vi "Initialize.vi"(8 "error in (no error)":errorcluster, 11 "UDP UI in":refnum<class "UDP User Interfaces.lvclass">) -> (0 "error out":errorcluster, 3 "UDP UI out":refnum<class "UDP User Interfaces.lvclass">)   [LabVIEW 2017, in "UDP User Interfaces.lvclass"]
uses:
  UDP User Interfaces.lvclass
  C:/Git/DSF/Core/Classes/Component User Interface/Component User Interfaces.lvclass
  Thread/UDP Thread User Interface.lvclass
  C:/Git/DSF/Core/Classes/User Interface/User Interface.lvclass
  Transfer Rx/UDP Transfer Rx User Interface.lvclass
  Transfer Tx/UDP Transfer Tx User Interface.lvclass
  Classes/Component User Interface/Component User Interfaces.lvclass
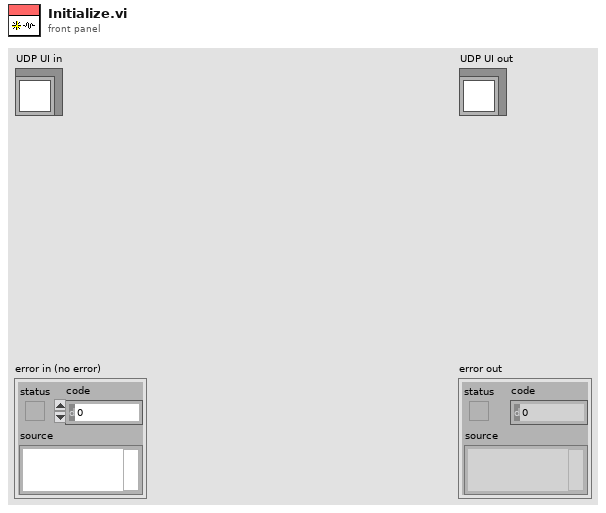
[diagram p1: front panel]
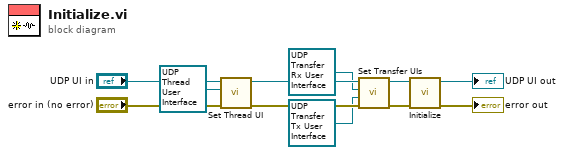
[diagram p0: block diagram]
diagram:
  n1 = call "Set Thread UI.vi"("error in (no error)"="error in (no error)", "Thread UI"=refnum<class "UDP Thread User Interface.lvclass"> refnum ("DSF Core.lvlib:UDP Thread UI.lvclass"), "Component UI in"="UDP UI in") -> ("error out"=w6:errorcluster, "Component UI out"=w5:refnum<class "UDP User Interfaces.lvclass">)  [unwired: 7 in]
  n2 = call "Set Transfer UIs.vi"("error in (no error)"=w6, "Tx Transfer UI"=refnum<class "UDP Transfer Tx User Interface.lvclass"> refnum ("DSF Core.lvlib:UDP Transfer Tx User Interface.lvclass"), "Rx Transfer UI"=refnum<class "UDP Transfer Rx User Interface.lvclass"> refnum ("DSF Core.lvlib:UDP Transfer Rx User Interface.lvclass"), "Component UI in"=w5) -> ("error out"=w1:errorcluster, "Component UI out"=w2:refnum<class "UDP User Interfaces.lvclass">)  [unwired: 6 in]
  n3 = call-parent "Initialize.vi"("error in (no error)"=w1, "Component UI in"=w2) -> ("error out"=→"error out":errorcluster, "Component UI out"=→"UDP UI out":refnum<class "UDP User Interfaces.lvclass">)  [unwired: 8 in]
